vi "CheckPause.vi"(3 "error in":errorcluster, 4 "Program (11)":u8=11 format="%.0x", 5 "Motion Board ID":u8 min=1 max=32 step=1) -> (0 "error out":errorcluster)   [LabVIEW 2022 SP3]
uses:
  <vilib>/Motion/FlexMotion/CustomControls/CustomControls.llb/Program.flx
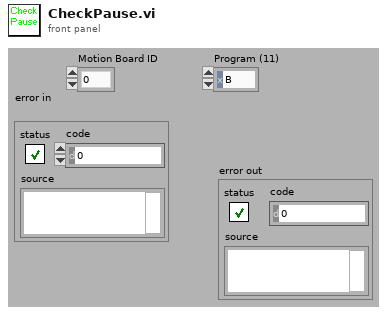
[diagram p1: front panel]
types:
  T1 = typedef "Program.flx" = u8
  T2 = typedef "Bd Id Out" = u8
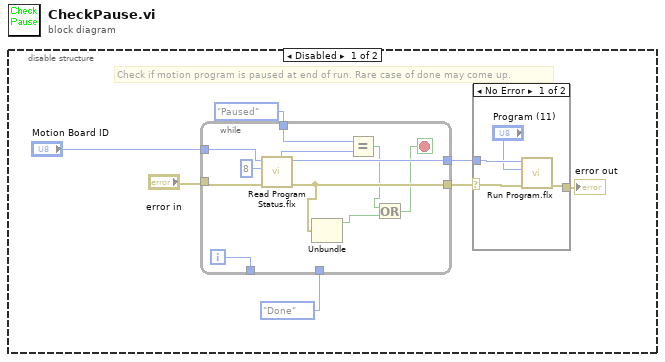
[diagram p0: block diagram]
diagram:
  n1 = disable-structure shown="Disabled" {
    frame Disabled {
      # "Check if motion program is paused at end of run. Rare case of done may come up."
      n2 = while {
        tunnel: [w22] -> w6
        tunnel: "error in" -> [w21]
        tunnel: [w17] -> w1
        tunnel: enum16{"Done", "Playing", "Paused", "Storing"}."Paused" ("Program Status") -> [w20]
        tunnel: "Motion Board ID" -> [w19]
        tunnel: enum16{"Done", "Playing", "Paused", "Storing"}."Done" ("Program Status") -> [_]
        tunnel: [w13] -> _
        i -> [w13]
        stop <- w14 stop-if-true
        n3 = call <vilib>:"Read Program Status.flx"("error in (no error)"=w21, "Program (1)"=T1 8, "Board Id"=w19) -> ("error out"=w17:errorcluster, "Bd Id Out"=w22:T2, "Program Status"=w18:enum16{"Done", "Playing", "Paused", "Storing"})  [unwired: 3 in, 1 out]
        n4 = Unbundle(w17) -> ("status"=w16:bool)  [unwired: 2 out]
        n5 = Equal?(x=w20, y=w18) -> (x = y?=w15:bool)
        n6 = Or(x=w15, y=w16) -> (x .or. y?=w14:bool)
      }
      n7 = case shown="No Error" w1 {
        selector: w1 -> [w8 w12]
        tunnel: w6 -> [w11 _]
        tunnel: [w10 w12] -> w5
        frame No Error {
          n8 = call <vilib>:"Run Program.flx"("error in (no error)"=w8, "Program (1)"="Program (11)", "Board ID"=w11) -> ("error out"=w10:errorcluster)  [unwired: 3 in, 2 out]
        }
        frame Error {
        }
      }
      "error out" <- w5
    }
    frame Enabled {
    }
  }
